vi "getAllRobotModelSamplesFromCSV.vi"(8 "error in (no error)":errorcluster, 11 "Utilities in":refnum<class "Utilities.lvclass">) -> (0 "error out":errorcluster, 3 "Utilities out":refnum<class "Utilities.lvclass">)   [LabVIEW 2023, in "Utilities.lvclass"]
uses:
  Utilities.lvclass
  Controls/RobotModel.ctl
panel:
  in  "last_triples_to_redo":dbl[][](array[numeric])=[[5.534782, 1.422991, 1.4, 274.0], [6.769919, 2.024429, 2.0, 385.0], [5.963033, 3.623179, 3.6, 661.0], [6.540693, 3.60129, 3.6, 664.0], [5.335392, 3.815569, 3.8, 693.0], [3.180777, 4.764794, 4.8, 858.0], [3.54737, 4.984863, 5.0, 895.0], [4.783766, 5.158272, 5.2, 936.0], [5.568159, 5.223424, 5.2, 939.0], [6.761975, 5.212306, 5.2, 945.0], [6.912103, 5.226409, 5.2, 946.0], [5.153213, 5.364369, 5.4, 973.0], [5.949899, 5.420473, 5.4, 976.0], [6.110103, 5.411127, 5.4, 977.0], [6.888686, 6.006165, 6.0, 1086.0], [4.348029, 6.366373, 6.4, 1144.0], [5.498483, 6.372701, 6.4, 1150.0], [1.339614, 6.574401, 6.6, 1164.0], [5.16234, 6.578302, 6.6, 1183.0], [4.94291, 6.75029, 6.8, 1217.0], [0.529303, 6.961511, 7.0, 1230.0], [1.326, 6.937678, 7.0, 1234.0], [1.764356, 6.960933, 7.0, 1236.0], [4.522583, 6.969642, 7.0, 1250.0], [4.938892, 6.967675, 7.0, 1252.0], [6.700275, 6.948454, 7.0, 1261.0], [6.6, 4.6, 4.6, 839.0]]
  out "min value":dbl
  out "max value":dbl
  out "size(s)":i32[](array[numeric])
  out "triples_to_redo":dbl[][](array[numeric])
  in  "all_samples path":path=path "C:/Users/RoboIme/git/sslview/Util/Farias2.csv"
  out "Array":T1[](array[typedef])
  in  "RobotModel":T1
  in  "std path":path=path "C:/Users/RoboIme/git/sslview/Util/Farias2.csv"
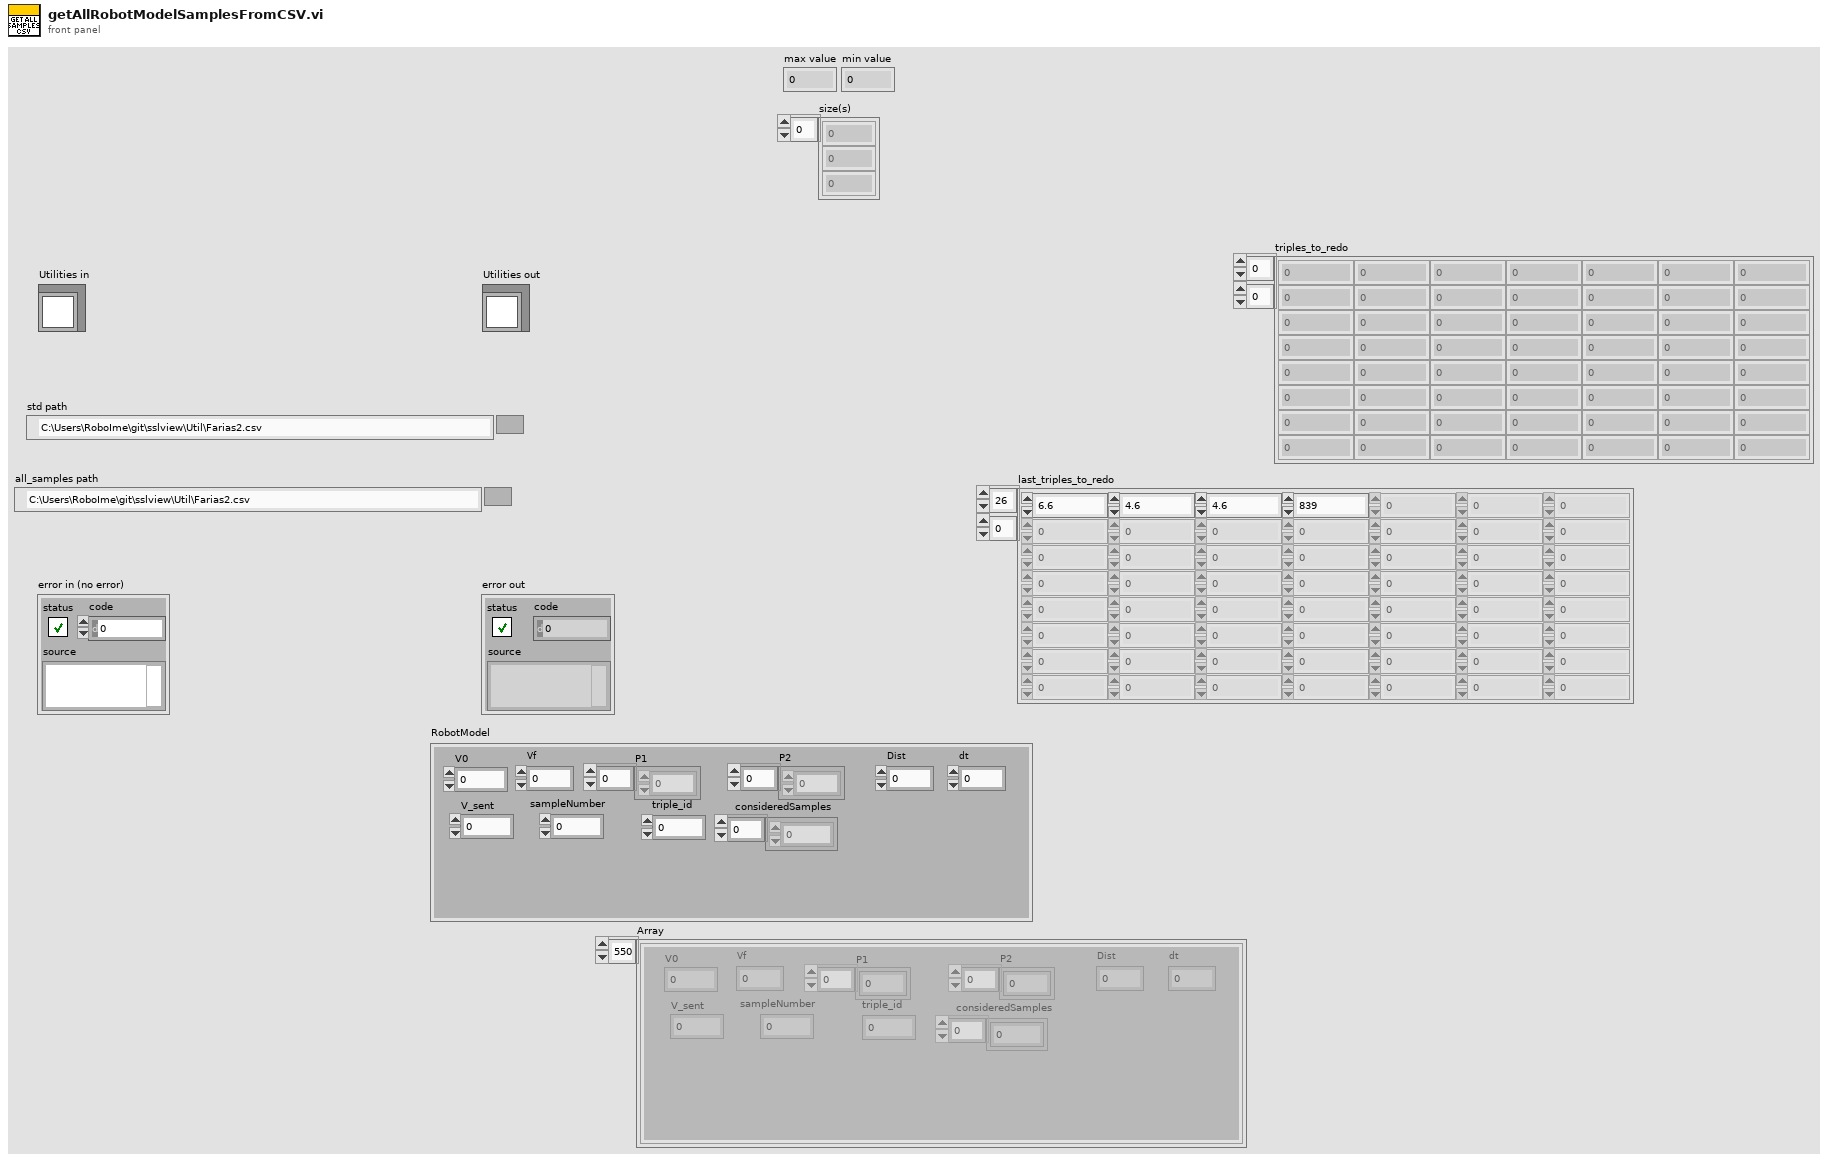
[diagram p1: front panel]
types:
  T1 = typedef "RobotModel.ctl" = cluster{"V0":dbl, "Vf":dbl, "Dist":dbl, "dt":dbl, "P1":dbl[], "P2":dbl[], "V_sent":dbl, "sampleNumber":i32, "triple_id":i32, "consideredSamples":dbl[]}
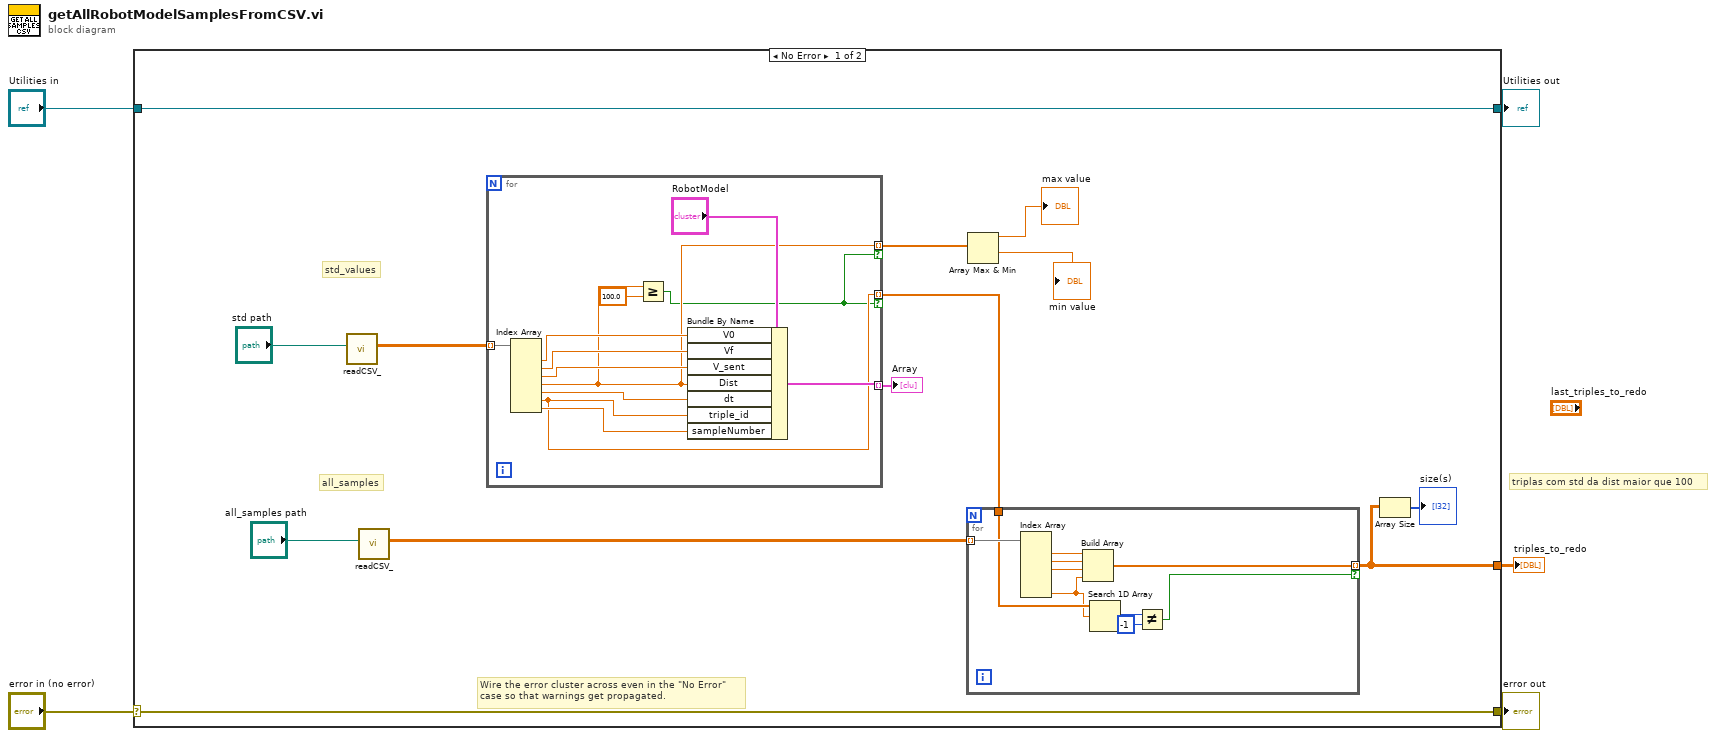
[diagram p0: block diagram]
diagram:
  # "triplas com std da dist maior que 100"
  n1 = case shown="No Error" "error in (no error)" {
    selector: "error in (no error)" -> [w17 w42]
    tunnel: [w17 w42] -> w4
    tunnel: [w18 w41] -> w2
    tunnel: "Utilities in" -> [w18 w41]
    tunnel: [w10 _] -> w1
    frame No Error {
      # "all_samples"
      # "std_values"
      # "Wire the error cluster across even in the \"No Error\"\ncase so that warnings get propagated."
      n2 = call "readCSV_.vi"("file path (use dialog)"="std path") -> ("array"=w15:dbl[][])  [unwired: 8 in, 2 out]
      n3 = call "readCSV_.vi"("file path (use dialog)"="all_samples path") -> ("array"=w12:dbl[][])  [unwired: 8 in, 2 out]
      n4 = for {
        tunnel: w15 -> [w40] mode=indexing
        tunnel: [w33] -> w14 mode=indexing
        tunnel: [w31] -> w11 mode=indexing if=w29
        tunnel: [w30] -> w8 mode=indexing if=w29
        n5 = Index Array(array=w40) -> (element #1=w38:dbl, element #2=w37:dbl, element #3=w36:dbl, element #4=w30:dbl, element #5=w35:dbl, element #6=w31:dbl, element #7=w34:dbl)  [unwired: 7 in]
        n6 = Greater Or Equal?(x=w30, y=100.0) -> (x >= y?=w29:bool)
        n7 = Bundle By Name(cluster="RobotModel", "V0"=w38, "Vf"=w37, "V_sent"=w36, "Dist"=w30, "dt"=w35, "triple_id"=w31, "sampleNumber"=w34) -> (w33:T1)
      }
      "Array" <- w14
      n8 = for {
        tunnel: w12 -> [w28] mode=indexing
        tunnel: [w25] -> w10 mode=indexing if=w20
        tunnel: w11 -> [w23]
        n9 = Index Array(array=w28) -> (element #1=w27:dbl, element #2=w26:dbl, element #3=w24:dbl, element #6=w19:dbl)  [unwired: 6 in, 2 out]
        n10 = Build Array(w27, w26, w24, w19) -> (w25:dbl[])
        n11 = Search 1D Array(1D array=w23, element=w19) -> (index of element=w22:i32)  [unwired: 1 in]
        n12 = Not Equal?(x=w22, y=-1) -> (x != y?=w20:bool)
      }
      n13 = Array Max & Min(array=w8) -> (max value=→"max value":dbl, min value=→"min value":dbl)  [unwired: 2 out]
      n14 = Array Size(array=w10) -> (size(s)=→"size(s)":i32[])
    }
    frame Error {
    }
  }
  "error out" <- w4
  "Utilities out" <- w2
  "triples_to_redo" <- w1
